vi "Diagnostic Logger v1.0.vi"   [LabVIEW 2014]
uses:
  <vilib>/Rock Robotics/WPI/DriverStation/WPI_DriverStationRobotMode2.ctl
  Begin/Global Variables.vi
  <vilib>/Utility/file.llb/Write To Spreadsheet File (DBL).vi
panel:
  # "CSV Columns Transposed:\n\nRobot Mode (0=?, 1=Auton, 2=Teleop)\nElapsed Time (ms)\ndt (ms)\nGyro Yaw\nGyro Pitch\nGyro Roll\nDriver JS LX\nDriver JS LY\nDriver JS RX\nDrive Resolver FL\nDrive Resolver FR\nDrive Resolver BL\nDrive Resolver BR\nDrive Encoder FL\nDrive Encoder FR\nDrive Encoder BL\nDrive Encoder BR\nDrive Speed FL\nDrive Speed FR\nDrive Speed BL\nDrive Speed BR\nLift Height Left\nLift Height Right\nLift Rate Left\nLift Rate Right"
  # "Data Usage Rates:\n\n20 KB / sec\n1.2 MB / min\n72 MB / hour"
types:
  T1 = typedef "WPI_DriverStationRobotMode2.ctl" = enum16{"Autonomous Disabled", "Autonomous Enabled", "Teleop Disabled", "Teleop Enabled", "Disconnected", "Finish", "Test Disabled", "Test Enabled", "Emergency Stopped"}
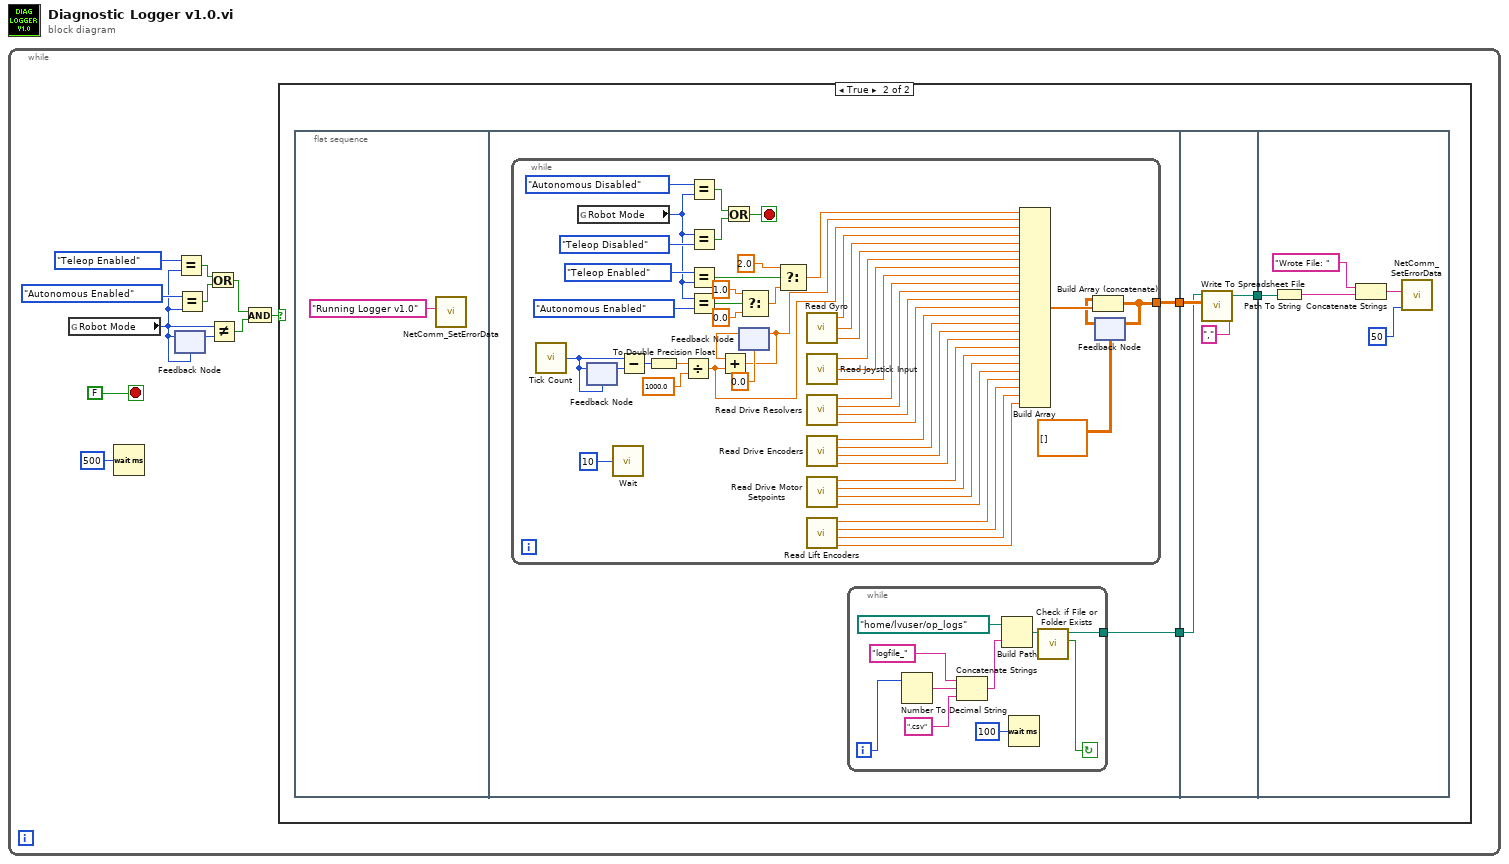
[diagram p0: block diagram]
diagram:
  n1 = while {
    stop <- FALSE stop-if-true
    n2 = global read "Global Variables.vi" "Robot Mode"() -> (w6:T1)
    n3 = Wait (ms)(milliseconds to wait=u32 500) -> ()  [unwired: 1 out]
    n4 = feedback-in #1(w6) -> ()
    n5 = feedback #1(w6) -> (w10:T1)
    n6 = Equal?(x=WPI_DriverStationRobotMode2."Teleop Enabled", y=w6) -> (x = y?=w5:bool)
    n7 = Equal?(x=WPI_DriverStationRobotMode2."Autonomous Enabled", y=w6) -> (x = y?=w4:bool)
    n8 = Or(x=w5, y=w4) -> (x .or. y?=w3:bool)
    n9 = Not Equal?(x=w6, y=w10) -> (x != y?=w9:bool)
    n10 = And(x=w3, y=w9) -> (x .and. y?=w2:bool)
    n11 = case shown="True" w2 {
      frame False {
      }
      frame True {
        n12 = flat-sequence {
          tunnel: [w17] -> w13
          tunnel: [w16] -> w12
          tunnel: [w81] -> w14
          tunnel: w13 -> [w80]
          tunnel: w12 -> [w79]
          tunnel: w14 -> [w83]
          frame #0 {
            n13 = call <vilib>:"NetComm_SetErrorData.vi"("Error Data"="Running Logger v1.0") -> ()  [unwired: 3 in, 8 out]
          }
          frame #1 {
            n14 = while {
              tunnel: [w30] -> w17
              stop <- w60 stop-if-true
              n15 = call "Tick Count"() -> ("Tick Count(uSec)"=w78:u32)
              n16 = global read "Global Variables.vi" "Robot Mode"() -> (w66:T1)
              n17 = feedback-in #2(w78) -> ()
              n18 = feedback #2(w78) -> (w77:u32)
              n19 = call "Wait"("Count(mSec)"=u32 10) -> ()  [unwired: 1 out]
              n20 = Subtract(x=w78, y=w77) -> (x-y=w59:u32)
              n21 = To Double Precision Float(number=w59) -> (double precision float=w58:dbl)
              n22 = Divide(x=w58, y=1000.0) -> (x/y=w54:dbl)
              n23 = Equal?(x=WPI_DriverStationRobotMode2."Autonomous Disabled", y=w66) -> (x = y?=w70:bool)
              n24 = Equal?(x=w66, y=WPI_DriverStationRobotMode2."Teleop Disabled" ("x")) -> (x = y?=w71:bool)
              n25 = Equal?(x=WPI_DriverStationRobotMode2."Teleop Enabled", y=w66) -> (x = y?=w68:bool)
              n26 = Equal?(x=w66, y=WPI_DriverStationRobotMode2."Autonomous Enabled" ("x")) -> (x = y?=w65:bool)
              n27 = Or(x=w70, y=w71) -> (x .or. y?=w60:bool)
              n28 = feedback #3(0.0) -> (w74:dbl)
              n29 = Add(x=w74, y=w54) -> (x+y=w55:dbl)
              n30 = feedback-in #3(w55) -> ()
              n31 = Select(t=1.0, s=w65, f=0.0) -> (s? t:f=w64:dbl)
              n32 = Select(t=2.0, s=w68, f=w64) -> (s? t:f=w56:dbl)
              n33 = call "Read Gyro.vi"() -> ("Roll"=w51:dbl, "Pitch"=w52:dbl, "Yaw"=w53:dbl)
              n34 = call "Read Joystick Input.vi"() -> ("Driver Joystick X2"=w48:dbl, "Driver Joystick Y1"=w49:dbl, "Driver Joystick X1"=w50:dbl)
              n35 = call "Read Drive Resolvers.vi"() -> ("Drive Resolver BR"=w44:dbl, "Drive Resolver BL"=w45:dbl, "Drive Resolver FR"=w46:dbl, "Drive Resolver FL"=w47:dbl)
              n36 = call "Read Drive Encoders.vi"() -> ("Drive Encoder BR"=w40:dbl, "Drive Encoder BL"=w41:dbl, "Drive Encoder FR"=w42:dbl, "Drive Encoder FL"=w43:dbl)
              n37 = call "Read Drive Motor Setpoints.vi"() -> ("Drive BR Setspeed"=w36:dbl, "Drive BL Setspeed"=w37:dbl, "Drive FR Setspeed"=w38:dbl, "Drive FL Setspeed"=w39:dbl)
              n38 = call "Read Lift Encoders.vi"() -> ("Lift Right Rate [counts/sec]"=w32:dbl, "Lift Left Rate [counts/sec]"=w33:dbl, "Lift Right Height [counts]"=w34:dbl, "Lift Left Height [counts]"=w35:dbl)
              n39 = Build Array(w56, w55, w54, w53, w52, w51, w50, w49, w48, w47, w46, w45, w44, w43, w42, w41, w40, w39, w38, w37, w36, w35, w34, w33, w32) -> (w31:dbl[])
              n40 = feedback #4(dbl[][] []) -> (w29:dbl[][])
              n41 = Build Array (concatenate)(w29, w31) -> (w30:dbl[][])
              n42 = feedback-in #4(w30) -> ()
            }
            n43 = while {
              tunnel: [w20] -> w16
              i -> [w19]
              stop <- w27 continue-if-true
              n44 = Number To Decimal String(number=w19) -> (decimal integer string=w24:string)  [unwired: 1 in]
              n45 = Concatenate Strings("logfile_", w24, ".csv") -> (w23:string)
              n46 = Build Path(base path=path "/home/lvuser/op_logs" ("file path (dialog if empty)"), name or relative path=w23) -> (appended path=w26:path)
              n47 = Wait (ms)(milliseconds to wait=u32 100) -> ()  [unwired: 1 out]
              n48 = call <vilib>:"Check if File or Folder Exists.vi"("path"=w26) -> ("file or folder exists?"=w27:bool, "dup path"=w20:path)  [unwired: 8 in, 1 out]
            }
          }
          frame #2 {
            n49 = call-poly <vilib>:"Write To Spreadsheet File.vi"("delimiter (\\t)"="," ("delimiter (\\t)"), "2D data"=w80, "file path (dialog if empty)"=w79) -> ("new file path (Not A Path if cancelled)"=w81:path)  [unwired: 5 in]
          }
          frame #3 {
            n50 = Path To String(path=w83) -> (string=w87:string)
            n51 = Concatenate Strings("Wrote File: ", w87) -> (w85:string)
            n52 = call <vilib>:"NetComm_SetErrorData.vi"("Timeout (ms)"=50, "Error Data"=w85) -> ()  [unwired: 2 in, 8 out]
          }
        }
      }
    }
  }
